vi "4.6.1.vi"(0 "停止":bool, 2 "数值 2":dbl, 3 "数值":dbl) -> (1 "x+y":dbl)   [LabVIEW 2017]
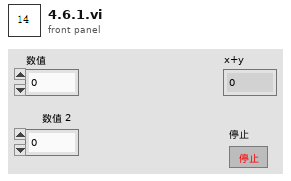
[diagram p1: front panel]
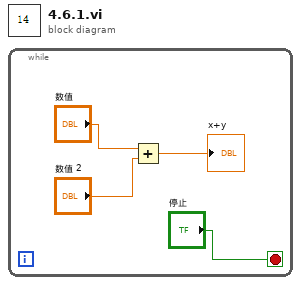
[diagram p0: block diagram]
diagram:
  n1 = while {
    stop <- "停止" stop-if-true
    n2 = Add(x="数值", y="数值 2") -> (x+y=→"x+y":dbl)
  }
